vi "get_y_cutoff_pixels.vi"(8 "error in (no error)":errorcluster, 11 "ImageAssemblerDL090211Frame in":refnum<class "ImageAssemblerDL090211Frame.lvclass">) -> (0 "error out":errorcluster, 2 "bottom cut-off":i32, 3 "ImageAssemblerDL090211Frame out":refnum<class "ImageAssemblerDL090211Frame.lvclass">, 5 "total lines per image":i32)   [LabVIEW 2010, in "ImageAssemblerDL090211Frame.lvclass"]
uses:
  ImageAssemblerDL090211Frame.lvclass
  ImageAssemblerDL090211Frame.lvclass/ImageAssemblerDL090211Frame.ctl
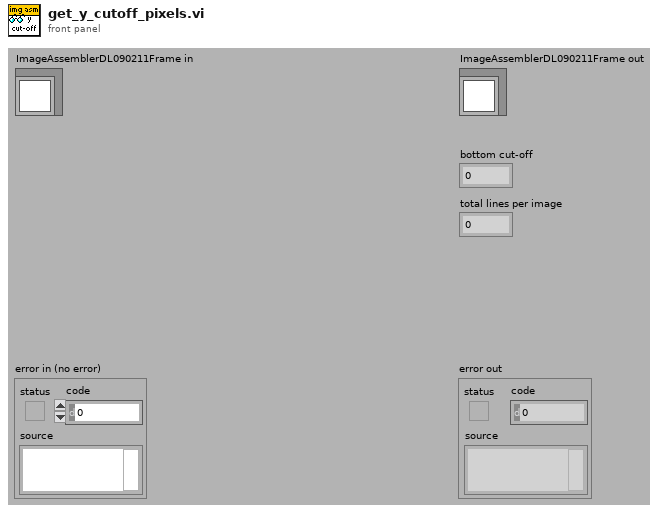
[diagram p1: front panel]
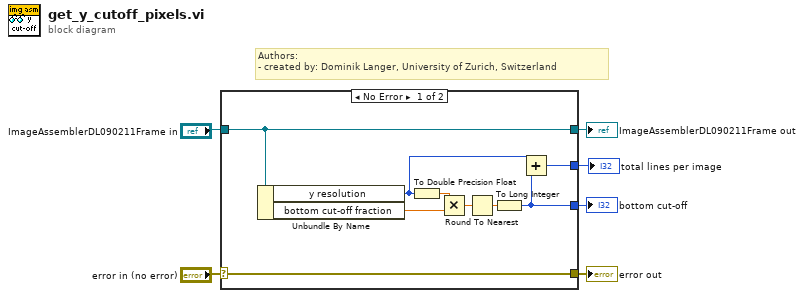
[diagram p0: block diagram]
diagram:
  # "Authors: \n- created by: Dominik Langer, University of Zurich, Switzerland"
  n1 = case shown="No Error" "error in (no error)" {
    selector: "error in (no error)" -> [w15 w17]
    tunnel: [w15 w17] -> w5
    tunnel: [w14 w16] -> w3
    tunnel: "ImageAssemblerDL090211Frame in" -> [w14 w16]
    tunnel: [w8 _] -> w2
    tunnel: [w7 _] -> w1
    frame No Error {
      n2 = Unbundle By Name(w14) -> ("y resolution"=w9:i32, "bottom cut-off fraction"=w12:dbl)
      n3 = To Double Precision Float(number=w9) -> (double precision float=w11:dbl)
      n4 = Multiply(x=w11, y=w12) -> (x*y=w10:dbl)
      n5 = Round To Nearest(number=w10) -> (nearest integer value=w13:dbl)
      n6 = To Long Integer(number=w13) -> (32bit integer=w8:i32)
      n7 = Add(x=w9, y=w8) -> (x+y=w7:i32)
    }
    frame Error {
    }
  }
  "error out" <- w5
  "ImageAssemblerDL090211Frame out" <- w3
  "bottom cut-off" <- w2
  "total lines per image" <- w1
